vi "ex2.vi"() -> ()   [LabVIEW 2017]
uses:
  <vilib>/sound2/lvsound2.llb/Sound Data Format.ctl
  <vilib>/sound2/lvsound2.llb/Sampling Mode.ctl
  <vilib>/sound2/lvsound2.llb/Sound File Write Open.vi
  <vilib>/sound2/lvsound2.llb/Sound Input Read (DBL).vi
  <vilib>/sound2/lvsound2.llb/Sound File Write (DBL).vi
panel:
  in  "path":path
  in  "stop":bool
  out "Time Signal":waveform(dbl)[](graph)
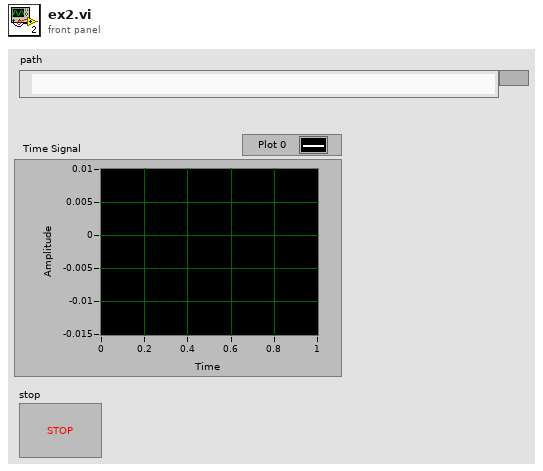
[diagram p1: front panel]
types:
  T1 = typedef "Sampling Mode.ctl" = i32
  T2 = typedef "Sound Data Format.ctl" = cluster{"sample rate (S/s)":dbl, "number of channels":i32, "bits per sample":i32}
  T3 = typedef "Sound Input Task ID.ctl" = u32
  T4 = typedef "Sound File Refnum.ctl" = refnum<file>
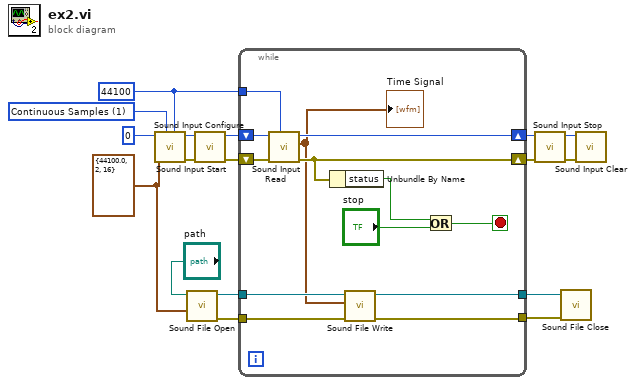
[diagram p0: block diagram]
diagram:
  w7 = 44100 ("number of samples/ch")
  w12 = T1 1 items=["Finite Samples", "Continuous Samples"] ("sample mode")
  w2 = T2 {"sample rate (S/s)"=44100.0, "number of channels"=2, "bits per sample"=16} ("sound format")
  n1 = call <vilib>:"Sound Input Configure.vi"("number of samples/ch"=w7, "sample mode"=w12, "sound format"=w2, "device ID"=u32 0) -> ("error out"=w16:errorcluster, "task ID"=w11:T3)  [unwired: 6 in]
  n2 = call-poly <vilib>:"Sound File Open.vi"("sound format"=w2, "path"="path") -> ("error out"=w6:errorcluster, "sound file refnum"=w4:T4)  [unwired: 8 in]
  n3 = call <vilib>:"Sound Input Start.vi"("error in (no error)"=w16, "task ID"=w11) -> ("error out"=w15:errorcluster, "task ID out"=w10:T3)  [unwired: 8 in]
  n4 = while {
    shift-right: [w27] -> w14
    shift-left: w15 -> [w30]
    shift-right: [w28] -> w8
    shift-left: w10 -> [w29]
    tunnel: w7 -> [w23]
    tunnel: w6 -> [w22]
    tunnel: [w21] -> w5
    tunnel: w4 -> [w20]
    tunnel: [w19] -> w3
    stop <- w24 stop-if-true
    n5 = call-poly <vilib>:"Sound Input Read.vi"("number of samples/ch"=w23, "error in (no error)"=w30, "task ID"=w29) -> ("error out"=w27:errorcluster, "data"=w18:waveform(dbl)[], "task ID out"=w28:T3)  [unwired: 6 in]
    "Time Signal" <- w18
    n6 = Unbundle By Name(w27) -> ("status"=w26:bool)
    n7 = call-poly <vilib>:"Sound File Write.vi"("error in (no error)"=w22, "data"=w18, "sound file refnum"=w20) -> ("error out"=w21:errorcluster, "sound file refnum out"=w19:T4)  [unwired: 7 in]
    n8 = Or(x=w26, y="stop") -> (x .or. y?=w24:bool)
  }
  n9 = call <vilib>:"Sound Input Stop.vi"("error in (no error)"=w14, "task ID"=w8) -> ("error out"=w13:errorcluster, "task ID out"=w9:T3)  [unwired: 8 in]
  n10 = call <vilib>:"Sound File Close.vi"("error in (no error)"=w5, "sound file refnum"=w3) -> ()  [unwired: 9 in, 1 out]
  n11 = call <vilib>:"Sound Input Clear.vi"("error in (no error)"=w13, "task ID"=w9) -> ()  [unwired: 9 in, 1 out]
